vi "SVI-Config-ReadWriteINIFile.vi"(6 "VI ref":refnum<vi>, 7 "Mode":enum16{"Read", "Write"}(ring), 8 "error in (no error)":errorcluster) -> (0 "error out":errorcluster, 3 "Path":path)   [LabVIEW 2024]
uses:
  <vilib>/Utility/config.llb/NI_LVConfig.lvlib
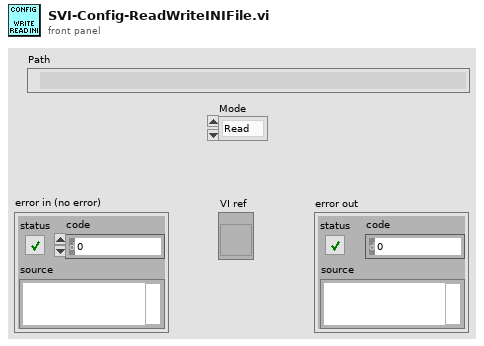
[diagram p1: front panel]
types:
  T1 = typedef "NI_LVConfig.lvlib/Config Data RefNum.ctl" = refnum<k1>
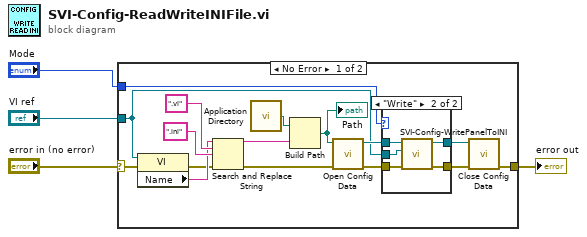
[diagram p0: block diagram]
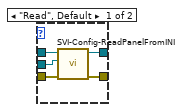
[diagram p2: hidden frame]
diagram:
  n1 = case shown="No Error" "error in (no error)" {
    selector: "error in (no error)" -> [w6 w31]
    tunnel: [w19 w31] -> w4
    tunnel: "Mode" -> [w13 _]
    tunnel: "VI ref" -> [w8 _]
    frame No Error {
      n2 = property class="VI"(reference=w8, error in=w6) -> (error out=w5:errorcluster, "Name"=w7:string)  [unwired: 1 out]
      n3 = Search and Replace String(input string=w7, search string=".vi", replace string=".ini" ("replace string (\"\")"), error in=w5) -> (result string=w10:string, error out=w9:errorcluster)  [unwired: 4 in, 2 out]
      n4 = call <vilib>:"Application Directory.vi"() -> ("Application Directory"=w20:path)
      n5 = Build Path(base path=w20, name or relative path=w10) -> (appended path=w18:path)
      "Path" <- w18
      n6 = call <vilib>:"Open Config Data.vi"("error in (no error)"=w9, "configuration file path"=w18) -> ("error out"=w16:errorcluster, "refnum"=w17:T1)  [unwired: 7 in, 1 out]
      n7 = case shown="\"Write\"" w13 {
        tunnel: w17 -> [w25 w30]
        tunnel: w16 -> [w22 w29]
        tunnel: [w21 w28] -> w15
        tunnel: [w23 w27] -> w14
        tunnel: w8 -> [w24 w26]
        frame "Read", Default {
          n8 = call "SVI-Config-ReadPanelFromINI.vi"("error in (no error)"=w22, "VI ref"=w24, "refnum"=w25) -> ("error out"=w21:errorcluster, "refnum out"=w23:T1)  [unwired: 7 in]
        }
        frame "Write" {
          n9 = call "SVI-Config-WritePanelToINI.vi"("error in (no error)"=w29, "VI ref"=w26, "refnum"=w30) -> ("error out"=w28:errorcluster, "refnum out"=w27:T1)  [unwired: 7 in]
        }
      }
      n10 = call <vilib>:"Close Config Data.vi"("error in (no error)"=w15, "refnum"=w14) -> ("error out"=w19:errorcluster)  [unwired: 8 in, 1 out]
    }
    frame Error {
    }
  }
  "error out" <- w4
